vi "Clock.vi"() -> (0 "Clock":bool)   [LabVIEW 2012]
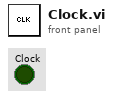
[diagram p1: front panel]
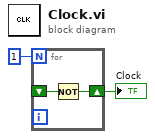
[diagram p0: block diagram]
diagram:
  n1 = for {
    N: 1 -> [_]
    shift-right: [w4] -> w2
    shift-left: _ -> [w3]
    n2 = Not(x=w3) -> (.not. x?=w4:bool)
  }
  "Clock" <- w2
